vi "URAPI Cmd.vi"(0 "BotSpeak CMD":string) -> (2 "Command":cluster{"CMD":string, "# params":i32}, 3 "Params":string)   [LabVIEW 2012]
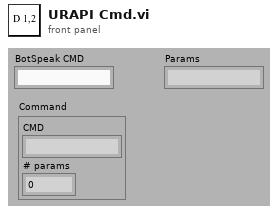
[diagram p1: front panel]
types:
  T1 = cluster{"result string":string, "number of replacements":i32}
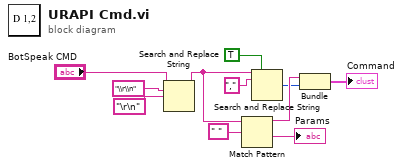
[diagram p0: block diagram]
diagram:
  n1 = Search and Replace String(input string="BotSpeak CMD", search string="\\r\\n" ("regular expression"), replace string="\r\n" ("regular expression")) -> (result string=w1:string)  [unwired: 5 in, 3 out]
  n2 = Match Pattern(string=w1, regular expression=" ") -> (before substring=w7:string, after substring=→"Params":string)  [unwired: 1 in, 2 out]
  n3 = Search and Replace String(replace all?=TRUE ("replace all? (F)"), input string=w1, search string="," ("regular expression")) -> (number of replacements=w6:i32)  [unwired: 5 in, 3 out]
  n4 = Bundle("result string"=w7, "number of replacements"=w6) -> (→"Command":T1)  [unwired: 1 in]
